vi "Loop.vi"(11 "Ex Event Actor in":refnum<class "Ex Event Actor.lvclass">) -> (3 "Ex Event Actor out":refnum<class "Ex Event Actor.lvclass">)   [LabVIEW 2021, in "Ex Event Actor.lvlib" / "Ex Event Actor.lvclass"]
uses:
  Ex Event Actor.lvclass
  Ex Event Actor.lvclass/Ex Event Actor.ctl
  Pop Up/Pop Up Msg/Pop Up Msg.lvclass
  Actor/Msgs/Teardown/Teardown Msg/Teardown Msg.lvclass
panel:
  in  "Button":bool
  out "String Indicator":string
  in  "Pop Up":bool
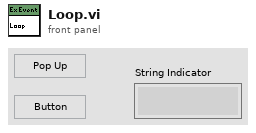
[diagram p1: front panel]
types:
  T1 = cluster{"Teardown":refnum<user-event>, "Pop Up":refnum<user-event>, "String Indicator":refnum<user-event>, "Button":refnum<user-event>}
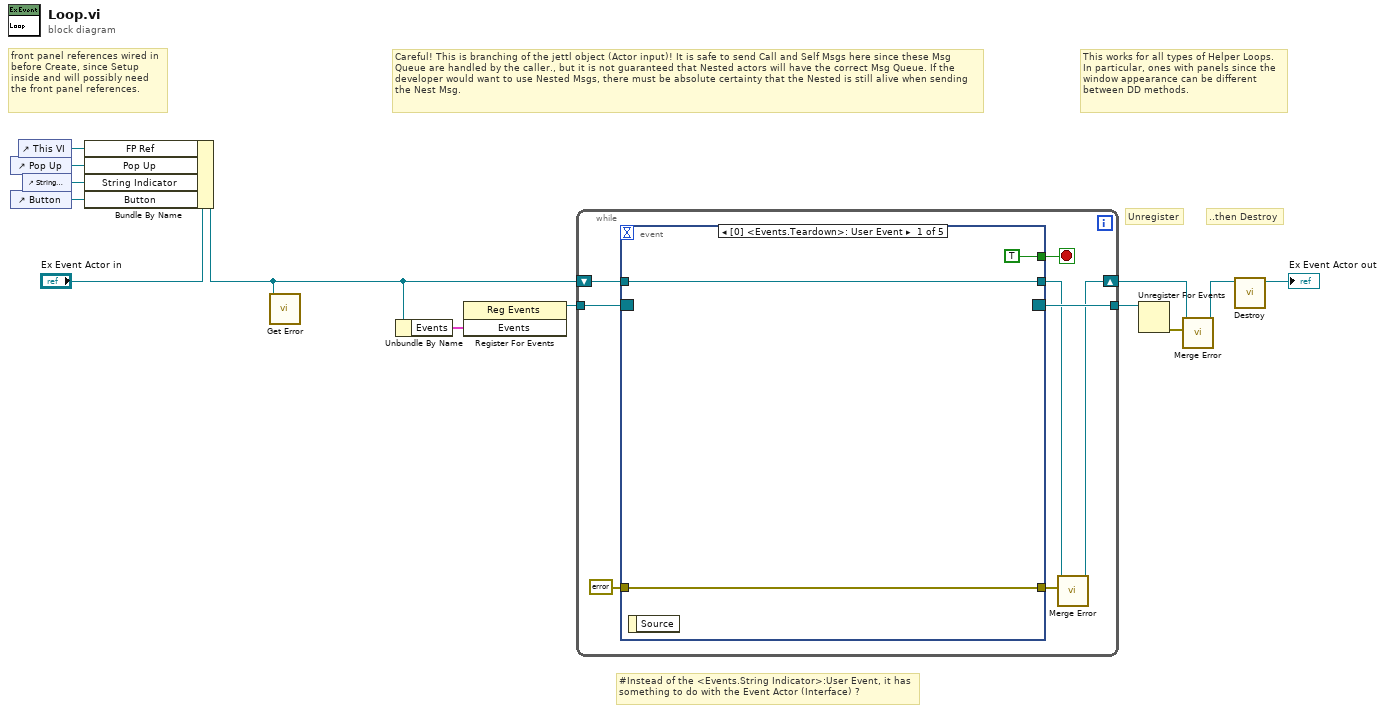
[diagram p0: block diagram]
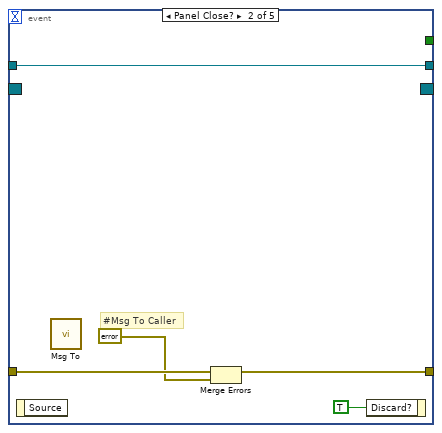
[diagram p2: hidden frame]
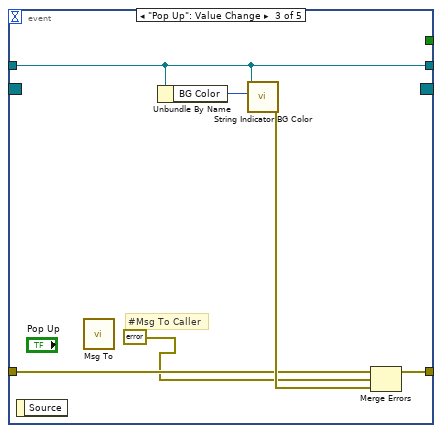
[diagram p3: hidden frame]
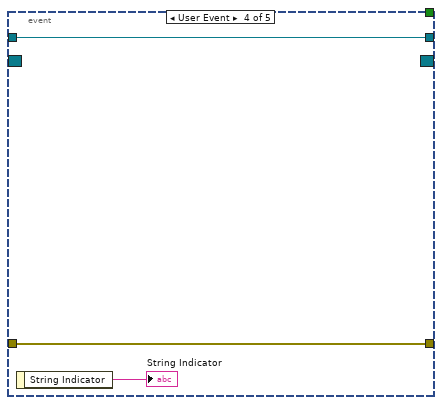
[diagram p4: hidden frame]
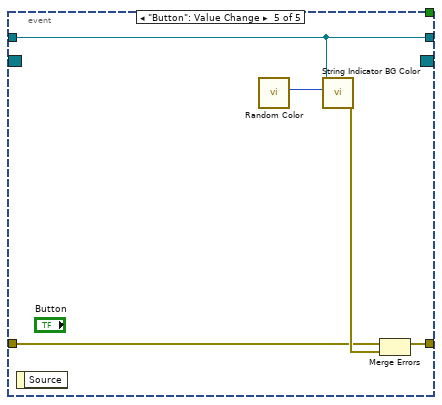
[diagram p5: hidden frame]
diagram:
  # "..then Destroy"
  # "Unregister"
  # "#Instead of the <Events.String Indicator>:User Event, it has something to do with the Event Actor (Interface) ?"
  # "front panel references wired in before Create, since Setup inside and will possibly need the front panel references."
  # "This works for all types of Helper Loops. In particular, ones with panels since the window appearance can be different between DD methods."
  # "Careful! This is branching of the jettl object (Actor input)! It is safe to send Call and Self Msgs here since these Msg Queue are handled by the caller., but it is not guaranteed that Nested actors will have the correct Msg Queue. If the developer would want to use Nested Msgs, there must be absolute certainty that the Nested is still alive when sending the Nest Msg."
  n1 = control-ref of="Pop Up"() -> (w12:refnum<vi>)
  n2 = control-ref of="Button"() -> (w11:refnum<vi>)
  n3 = control-ref of="This VI"() -> (w10:refnum<vi>)
  n4 = control-ref of="String Indicator"() -> (w13:refnum<vi>)
  n5 = Bundle By Name(cluster="Ex Event Actor in", "FP Ref"=w10, "Pop Up"=w12, "String Indicator"=w13, "Button"=w11) -> (w8:refnum<class "Ex Event Actor.lvclass">)
  n6 = call-dynamic "Get Error.vi"("Ex Event Actor in"=w8) -> ()  [unwired: 10 in, 1 out]
  n7 = Unbundle By Name(w8) -> ("Events"=w4:T1)
  n8 = register-events ("Main Register for Events")(w4) -> (reference out=w5:refnum<event-registration>)  [unwired: 2 in, 1 out]
  n9 = while {
    shift-right: [w16] -> w3
    shift-left: w8 -> [w18]
    tunnel: w5 -> [w21]
    tunnel: [w19] -> w6
    stop <- w20 stop-if-true
    n10 = event "UI Events" shown="[0] <Events.Teardown>: User Event" {
      selector: w21 -> [_ _ _ _ _]
      dyn-events: [_ _ _ _ _] -> w19
      timeout: _ -> [_ _ _ _ _]
      tunnel: [TRUE _ _ _ _] -> w20
      tunnel: [w23 w26 w31 w38 w43] -> w17
      tunnel: w18 -> [w23 w26 w31 w38 w43]
      tunnel: [w22 w28 w35 w37 w42] -> w15
      tunnel: errorcluster {"status"=FALSE, "code"=0, "source"=""} ("error out") -> [w22 w27 w32 w37 w40]
      event User Event {
        n11 = event-data() -> ()  [unwired: 1 in, 1 out]
      }
      event Panel Close? {
        # "#Msg To Caller"
        n12 = event-data() -> ()  [unwired: 1 in, 1 out]
        n13 = call "Msg To.vi"() -> ()  [unwired: 11 in, 1 out]
        n14 = Merge Errors(w27, errorcluster {"status"=FALSE, "code"=0, "source"=""} ("error in")) -> (w28:errorcluster)
        n15 = event-data("Discard?"=TRUE) -> ()  [unwired: 1 in, 1 out]
      }
      event "Pop Up": Value Change {
        # "#Msg To Caller"
        n16 = event-data() -> ()  [unwired: 1 in, 1 out]
        n17 = call "Msg To.vi"() -> ()  [unwired: 11 in, 1 out]
        n18 = Unbundle By Name(w31) -> ("BG Color"=w33:u32)
        n19 = call "String Indicator BG Color.vi"("BG Color"=w33, "Ex Event Actor in"=w31) -> ("error out"=w34:errorcluster)  [unwired: 9 in]
        n20 = Merge Errors(w32, errorcluster {"status"=FALSE, "code"=0, "source"=""} ("error in"), w34) -> (w35:errorcluster)
      }
      event User Event {
        n21 = event-data() -> ("String Indicator"=→"String Indicator":string)  [unwired: 1 in]
      }
      event "Button": Value Change {
        n22 = event-data() -> ()  [unwired: 1 in, 1 out]
        n23 = call "Random Color.vi"() -> ("Color"=w39:u32)  [unwired: 11 in]
        n24 = call "String Indicator BG Color.vi"("BG Color"=w39, "Ex Event Actor in"=w43) -> ("error out"=w41:errorcluster)  [unwired: 9 in]
        n25 = Merge Errors(w40, w41) -> (w42:errorcluster)
      }
    }
    n26 = call-dynamic "Merge Error.vi"("Error"=w15, "Ex Event Actor in"=w17) -> ("Ex Event Actor out"=w16:refnum<class "Ex Event Actor.lvclass">)  [unwired: 9 in]
  }
  n27 = Unregister For Events(event registration refnum=w6) -> (error out=w2:errorcluster)  [unwired: 1 in]
  n28 = call-dynamic "Merge Error.vi"("Error"=w2, "Ex Event Actor in"=w3) -> ("Ex Event Actor out"=w1:refnum<class "Ex Event Actor.lvclass">)  [unwired: 9 in]
  n29 = call-dynamic "Destroy.vi"("Ex Event Actor in"=w1) -> ("Ex Event Actor out"=→"Ex Event Actor out":refnum<class "Ex Event Actor.lvclass">)  [unwired: 10 in]
